vi "ESA-C Live Control.vi"(1 "Running":refnum<vi>, 3 "Drive Live Controls":T1={"Snapshot"=FALSE, "Move Step"=1.0, "Move Home"=FALSE, "Move Down"=FALSE, "Move Up"=FALSE, "Move Left"=FALSE, "Move Right"=FALSE, "Move Out"=FALSE, "Move In"=FALSE} {"Move Step" min=0.0 max=30.0 step=0.1 format="%.1f"}, 4 "Drive Connection Settings":T2={"Objective GPIB-Port"=4, "Stage GPIB-Port"=4, "Drive Selector"=0, "Drive Velocity (V/s)"=5.0} {"Drive Velocity (V/s)" min=10.0 max=160.0 step=0.1 format="%.1f"; "Drive Selector" items=["Obj.", "Stage"]; "Stage GPIB-Port" min=1 max=20 step=1 format="%#.0f"; "Objective GPIB-Port" min=1 max=20 step=1 format="%#.0f"}) -> (0 "Reset Switches":bool)   [LabVIEW 2010]
uses:
  TypeDefs/ESA-C Connection Settings.ctl
  TypeDefs/ESA-C Live Controls.ctl
panel:
  # "XY"
  # "Z"
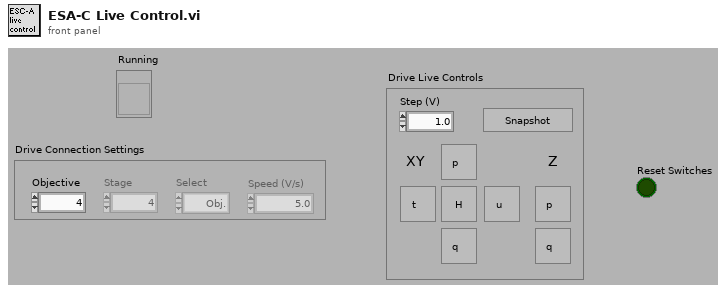
[diagram p1: front panel]
types:
  T1 = typedef "ESA-C Live Controls.ctl" = cluster{"Snapshot":bool, "Move Step":dbl, "Move Home":bool, "Move Down":bool, "Move Up":bool, "Move Left":bool, "Move Right":bool, "Move Out":bool, "Move In":bool}
  T2 = typedef "ESA-C Connection Settings.ctl" = cluster{"Objective GPIB-Port":i32, "Stage GPIB-Port":i32, "Drive Selector":u16, "Drive Velocity (V/s)":dbl}
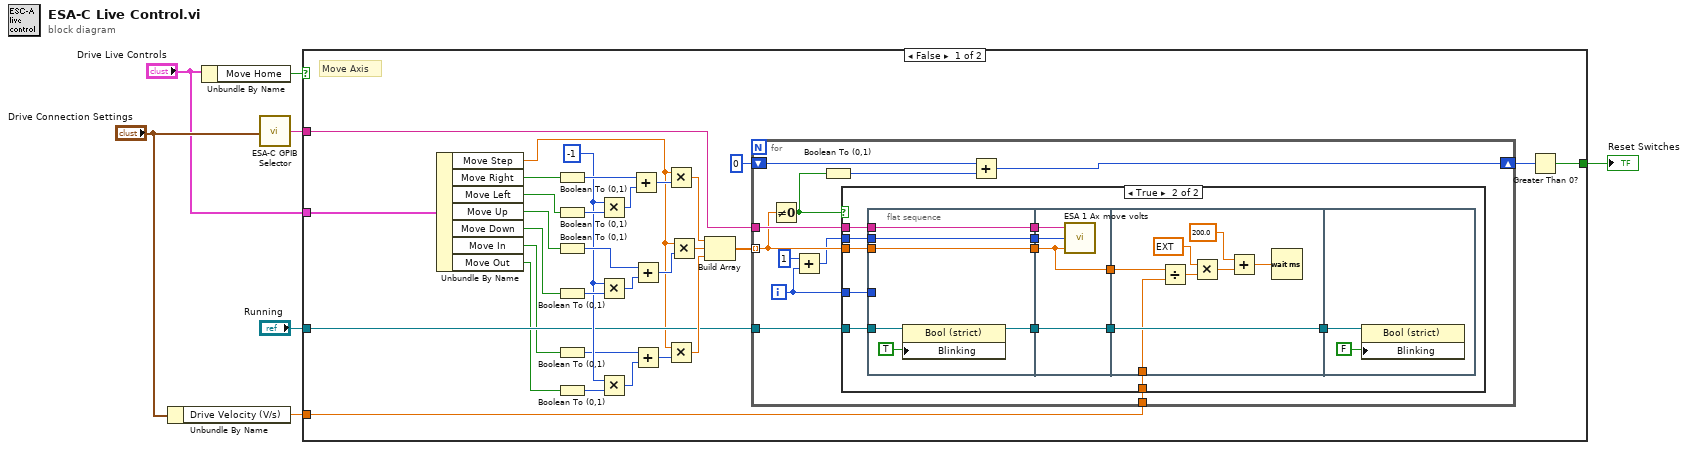
[diagram p0: block diagram]
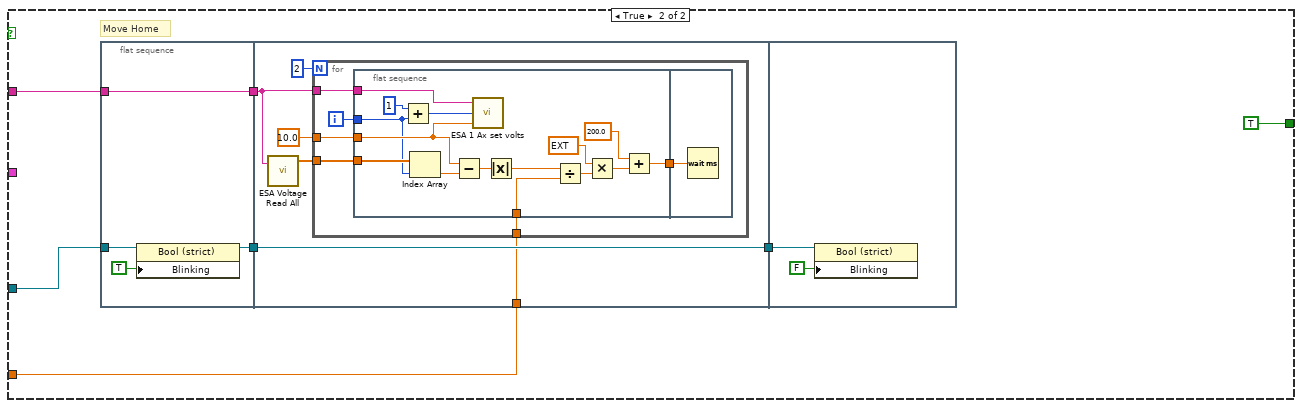
[diagram p3: hidden frame]
diagram:
  n1 = Unbundle By Name("Drive Connection Settings") -> ("Drive Velocity (V/s)"=w3:dbl)
  n2 = Unbundle By Name("Drive Live Controls") -> ("Move Home"=w1:bool)
  n3 = call "ESA-C GPIB Selector.vi"("Drive Connection Settings"="Drive Connection Settings") -> ("String"=w5:string)
  n4 = case shown="False" w1 {
    tunnel: w5 -> [w27 w88]
    tunnel: [w25 TRUE ("Reset Switches")] -> w7
    tunnel: "Running" -> [w17 w86]
    tunnel: w3 -> [w16 w83]
    tunnel: "Drive Live Controls" -> [w8 _]
    frame False {
      w22 = -1
      # "Move Axis"
      n5 = Unbundle By Name(w8) -> ("Move Step"=w9:dbl, "Move Right"=w10:bool, "Move Left"=w15:bool, "Move Up"=w14:bool, "Move Down"=w13:bool, "Move In"=w12:bool, "Move Out"=w11:bool)
      n6 = Boolean To (0,1)(Boolean=w10) -> (0, 1=w30:i16)
      n7 = Boolean To (0,1)(Boolean=w15) -> (0, 1=w28:i16)
      n8 = Boolean To (0,1)(Boolean=w14) -> (0, 1=w32:i16)
      n9 = Boolean To (0,1)(Boolean=w13) -> (0, 1=w29:i16)
      n10 = Boolean To (0,1)(Boolean=w12) -> (0, 1=w20:i16)
      n11 = Boolean To (0,1)(Boolean=w11) -> (0, 1=w23:i16)
      n12 = Multiply(x=w22, y=w28) -> (x*y=w31:i32)
      n13 = Multiply(x=w22, y=w29) -> (x*y=w33:i32)
      n14 = Multiply(x=w22, y=w23) -> (x*y=w21:i32)
      n15 = Add(x=w30, y=w31) -> (x+y=w34:i32)
      n16 = Add(x=w32, y=w33) -> (x+y=w35:i32)
      n17 = Add(x=w20, y=w21) -> (x+y=w19:i32)
      n18 = Multiply(x=w9, y=w34) -> (x*y=w36:dbl)
      n19 = Multiply(x=w9, y=w19) -> (x*y=w18:dbl)
      n20 = Multiply(x=w9, y=w35) -> (x*y=w37:dbl)
      n21 = Build Array(w36, w37, w18) -> (w38:dbl[])
      n22 = for {
        tunnel: w38 -> [w48] mode=indexing
        tunnel: w27 -> [w49]
        shift-right: [w44] -> w26
        shift-left: i16 0 -> [w45]
        tunnel: w17 -> [w41]
        tunnel: w16 -> [w40]
        i -> [w39]
        n23 = Not Equal To 0?(x=w48) -> (x != 0?=w47:bool)
        n24 = Add(x=1, y=w39) -> (x+y=w42:i32)
        n25 = Boolean To (0,1)(Boolean=w47) -> (0, 1=w46:i16)
        n26 = case shown="True" w47 {
          tunnel: w48 -> [_ w60]
          tunnel: w49 -> [_ w62]
          tunnel: w42 -> [_ w61]
          tunnel: w41 -> [_ w56]
          tunnel: w40 -> [_ w52]
          tunnel: w39 -> [_ w50]
          frame False {
          }
          frame True {
            n27 = flat-sequence {
              tunnel: w60 -> [w63]
              tunnel: w61 -> [w67]
              tunnel: w62 -> [w68]
              tunnel: [w68] -> w58
              tunnel: [w67] -> w57
              tunnel: w56 -> [w65]
              tunnel: [w64] -> w53
              tunnel: [w63] -> w51
              tunnel: w50 -> [_]
              tunnel: [w69] -> w59
              tunnel: w58 -> [w72]
              tunnel: w57 -> [w71]
              tunnel: [w70] -> w54
              tunnel: w53 -> [w70]
              tunnel: w51 -> [w69]
              tunnel: w59 -> [w75]
              tunnel: [w80] -> w55
              tunnel: w54 -> [w80]
              tunnel: w52 -> [w73]
              tunnel: w55 -> [w81]
              frame #0 {
                n28 = property class="Bool (strict)"(reference=w65, "Blinking"=TRUE ("Blinkend")) -> (reference out=w64:refnum<vi>)  [unwired: 1 in, 1 out]
              }
              frame #1 {
                n29 = call "ESA 1 Ax move volts.vi"("Voltage"=w69, "Axis"=w71, "GPIB Add"=w72) -> ()
              }
              frame #2 {
                n30 = Divide(x=w75, y=w73) -> (x/y=w76:dbl)
                n31 = Multiply(x=ext 1000.0, y=w76) -> (x*y=w79:ext)
                n32 = Add(x=200.0, y=w79) -> (x+y=w74:ext)
                n33 = Wait (ms)(milliseconds to wait=w74) -> ()  [unwired: 1 out]
              }
              frame #3 {
                n34 = property class="Bool (strict)"(reference=w81, "Blinking"=FALSE ("Blinkend")) -> ()  [unwired: 1 in, 2 out]
              }
            }
          }
        }
        n35 = Add(x=w45, y=w46) -> (x+y=w44:i16)
      }
      n36 = Greater Than 0?(x=w26) -> (x > 0?=w25:bool)
    }
    frame True {
      # "Move Home"
      n37 = flat-sequence {
        tunnel: w88 -> [w93]
        tunnel: [w93] -> w87
        tunnel: w86 -> [w91]
        tunnel: [w90] -> w84
        tunnel: w87 -> [w97]
        tunnel: [w95] -> w85
        tunnel: w84 -> [w95]
        tunnel: w83 -> [w94]
        tunnel: w85 -> [w122]
        frame #0 {
          n38 = property class="Bool (strict)"(reference=w91, "Blinking"=TRUE ("Blinkend")) -> (reference out=w90:refnum<vi>)  [unwired: 1 in, 1 out]
        }
        frame #1 {
          n39 = call "ESA Voltage Read All.vi"("GPIB Addr"=w97) -> ("Voltages"=w96:dbl[])  [unwired: 3 in]
          n40 = for {
            N: 2 -> [_]
            tunnel: 10.0 ("Voltage") -> [w102]
            tunnel: w97 -> [w104]
            tunnel: w96 -> [w103]
            tunnel: w94 -> [w100]
            i -> [w101]
            n41 = flat-sequence {
              tunnel: [w106] -> w105
              tunnel: w104 -> [w116]
              tunnel: w103 -> [w115]
              tunnel: w102 -> [w114]
              tunnel: w101 -> [w113]
              tunnel: w100 -> [w108]
              tunnel: w105 -> [w121]
              frame #0 {
                n42 = Add(x=1, y=w113) -> (x+y=w118:i32)
                n43 = Index Array(array=w115, index=w113) -> (element=w120:dbl)
                n44 = Subtract(x=w114, y=w120) -> (x-y=w119:dbl)
                n45 = call "ESA 1 Ax set volts.vi"("Voltage"=w114, "Axis"=w118, "GPIB Add"=w116) -> ()
                n46 = Absolute Value(x=w119) -> (abs(x)=w107:dbl)
                n47 = Divide(x=w107, y=w108) -> (x/y=w112:dbl)
                n48 = Multiply(x=ext 1000.0, y=w112) -> (x*y=w109:ext)
                n49 = Add(x=200.0, y=w109) -> (x+y=w106:ext)
              }
              frame #1 {
                n50 = Wait (ms)(milliseconds to wait=w121) -> ()  [unwired: 1 out]
              }
            }
          }
        }
        frame #2 {
          n51 = property class="Bool (strict)"(reference=w122, "Blinking"=FALSE ("Blinkend")) -> ()  [unwired: 1 in, 2 out]
        }
      }
    }
  }
  "Reset Switches" <- w7
